vi "SSC Digital Select Function.vi"(0 "Digital SSC in":T1[](array[typedef]), 5 "Function":T2=1100 items=["Digital"=1100, "PPMU"=1101, "Off"=1102, "Disconnect"=1103], 11 "error in":errorcluster) -> (4 "Digital SSC out":T1[](array[typedef]), 15 "error out":errorcluster)   [LabVIEW 2020]
doc: "Specifies whether digital pattern instruments connected to the specified pin(s) and pin group(s) are controlled by the PPMU, Digital, disconnected, or off. Changes take effect immediately."
uses:
  <instrlib>/niDigital/niDigital.llb/niDigital Selected Function.ctl
  SSC Digital.ctl
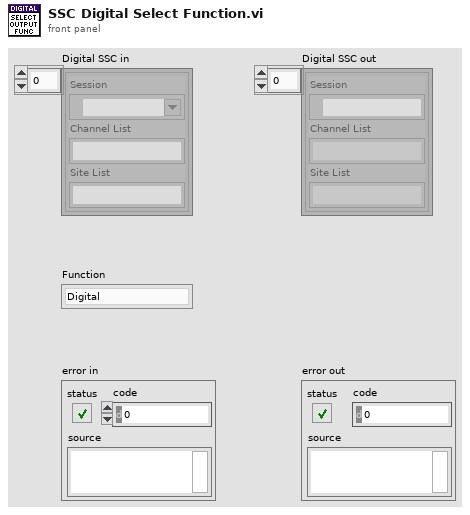
[diagram p1: front panel]
types:
  T1 = typedef "SSC Digital.ctl" = cluster{"Session":refnum<k15>, "Channel List":string, "Site List":string}
  T2 = typedef "niDigital Selected Function.ctl" = i32
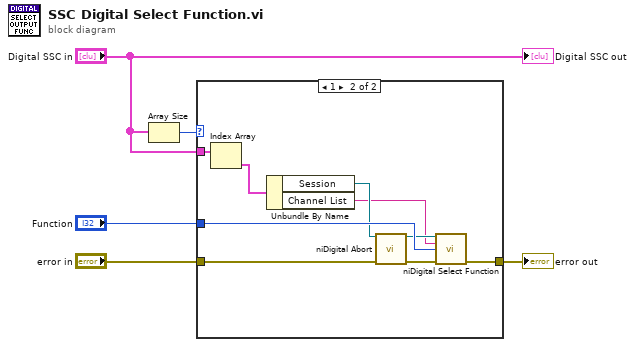
[diagram p0: block diagram]
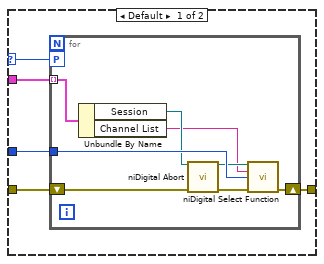
[diagram p2: hidden frame]
diagram:
  n1 = Array Size(array="Digital SSC in") -> (size(s)=w2:i32)
  n2 = case shown="1" w2 {
    selector: w2 -> [w7 _]
    tunnel: "Function" -> [w10 w27]
    tunnel: "error in" -> [w9 w26]
    tunnel: [w8 w25] -> w3
    tunnel: "Digital SSC in" -> [w6 w24]
    frame Default {
      n3 = for {
        tunnel: w10 -> [w17]
        workers-P: w7 -> [_]
        tunnel: w6 -> [w13] mode=indexing
        shift-right: [w18] -> w8
        shift-left: w9 -> [w16]
        n4 = Unbundle By Name(w13) -> ("Session"=w12:refnum<k15>, "Channel List"=w11:string)
        n5 = call <instrlib>:"niDigital Abort.vi"("instrument handle"=w12, "error in"=w16) -> ("instrument handle out"=w14:refnum<k15>, "error out"=w15:errorcluster)  [unwired: 12 in]
        n6 = call <instrlib>:"niDigital Select Function.vi"("instrument handle"=w14, "channel list"=w11, "function"=w17, "error in"=w15) -> ("error out"=w18:errorcluster)  [unwired: 10 in, 1 out]
      }
    }
    frame 1 {
      n7 = Index Array(array=w24) -> (element=w19:T1)  [unwired: 1 in]
      n8 = Unbundle By Name(w19) -> ("Session"=w21:refnum<k15>, "Channel List"=w20:string)
      n9 = call <instrlib>:"niDigital Abort.vi"("instrument handle"=w21, "error in"=w26) -> ("instrument handle out"=w22:refnum<k15>, "error out"=w23:errorcluster)  [unwired: 12 in]
      n10 = call <instrlib>:"niDigital Select Function.vi"("instrument handle"=w22, "channel list"=w20, "function"=w27, "error in"=w23) -> ("error out"=w25:errorcluster)  [unwired: 10 in, 1 out]
    }
  }
  "error out" <- w3
  "Digital SSC out" <- "Digital SSC in"
